vi "from string array.vi"(8 "error in (no error)":errorcluster, 9 "String Array":string[][](array[string]), 10 "version":string, 11 "module configuration in":refnum<class "SystemLink configuration.lvclass">) -> (0 "error out":errorcluster, 3 "module configuration out":refnum<class "SystemLink configuration.lvclass">)   [LabVIEW 2015, in "SystemLink configuration.lvclass"]
uses:
  SystemLink configuration.lvclass
  <vilib>/NI/Tag Bus Module Framework/channel/TBM channel.lvclass
  permissions.ctl
  <vilib>/NI/Tag Bus/tag/Data Type.ctl
  <vilib>/NI/Tag Bus/tag/tag descriptor.lvclass
  Line.ctl
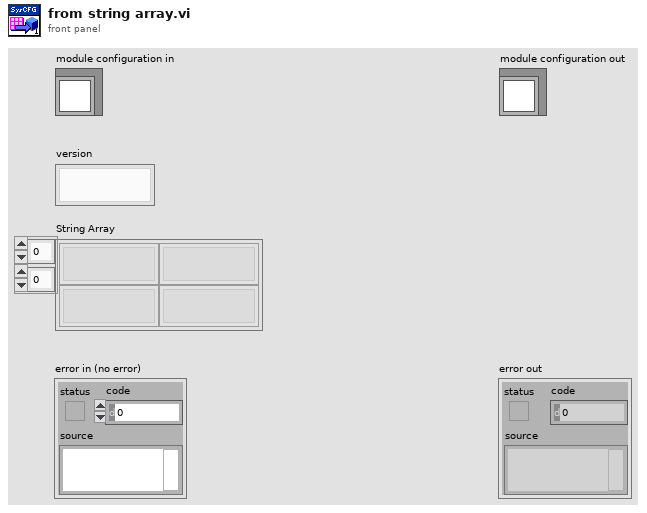
[diagram p1: front panel]
types:
  T1 = typedef "SystemLink configuration.lvclass/Line.ctl" = cluster{"channel":refnum<class "TBM channel.lvclass">, "Data Tag Type":enum16{"Double", "Single", "I32", "I16", "I8", "U64", "U32", "U16", "U8", "Boolean", "String", "Timestamp"}}
  T2 = typedef "tag bus.lvlib/tag descriptor.lvclass/Data Type.ctl" = enum16{"Double", "Single", "I64", "I32", "I16", "I8", "U64", "U32", "U16", "U8", "Boolean", "String", "Array of Double", "Array of Single", "Array of I64", "Array of I32", "Array of I16", "Array of I8", "Array of U64", "Array of U32", "Array of U16", "Array of U8", "Array of Boolean", "Array of String"}
  T3 = typedef "SystemLink configuration.lvclass/permissions.ctl" = enum32{"Read from SystemLink", "Write to SystemLink"}
  T4 = typedef "TBM channel.lvclass/channel classification.ctl" = enum16{"input data", "output data", "processing parameter", "processing result"}
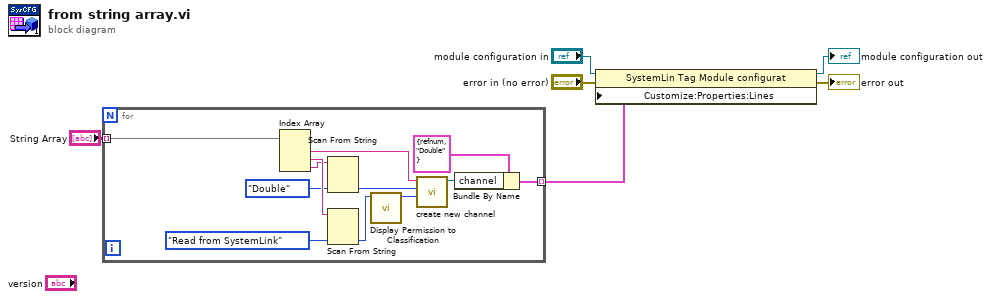
[diagram p0: block diagram]
diagram:
  n1 = for {
    tunnel: "String Array" -> [w18] mode=indexing
    tunnel: [w7] -> w1 mode=indexing
    n2 = Index Array(array=w18) -> (element #1=w17:string, element #2=w13:string, element #3=w12:string)  [unwired: 3 in]
    n3 = Scan From String(input string=w12, default 1=Data_Type."Double" ("data type")) -> (output 1=w10:T2)  [unwired: 3 in, 3 out]
    n4 = Scan From String(input string=w13, default 1=permissions."Read from SystemLink" ("display permissions")) -> (output 1=w15:T3)  [unwired: 3 in, 3 out]
    n5 = call "Display Permission to Classification.vi"("display permissions"=w15) -> ("channel classification"=w14:T4)  [unwired: 10 in]
    n6 = call <vilib>:"create new channel.vi"("channel classification"=w14, "data type"=w10, "channel name"=w17) -> ("channel"=w8:refnum<class "TBM channel.lvclass">)  [unwired: 8 in]
    n7 = Bundle By Name(cluster=T1 {"channel"=refnum, "Data Tag Type"=enum."Double"} ("Line"), "channel"=w8) -> (w7:T1)
  }
  n8 = property class="SystemLin Tag Module configurat"(reference="module configuration in", error in="error in (no error)", "Customize:Properties:Lines"=w1) -> (reference out=→"module configuration out":refnum<class "SystemLink configuration.lvclass">, error out=→"error out":errorcluster)
